vi "TableToArray(SubVI).vi"(11 "String in":string) -> (2 "Array":sgl[](array[numeric]))   [LabVIEW 2017, in "LV_Unicorn.lvlib"]
uses:
  LV_Unicorn.lvlib
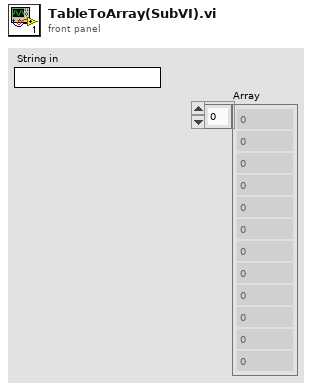
[diagram p1: front panel]
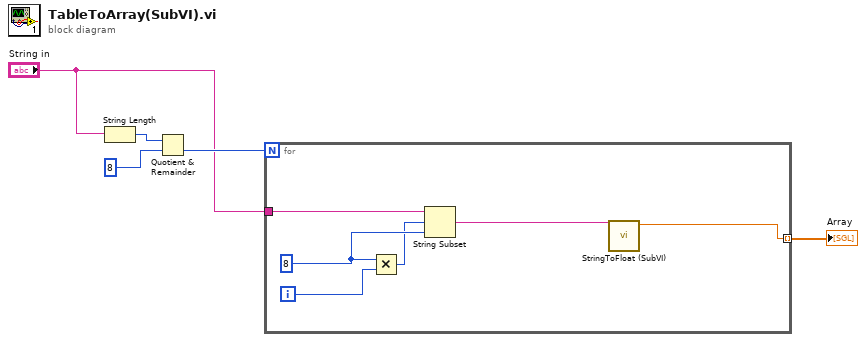
[diagram p0: block diagram]
diagram:
  n1 = String Length(string="String in") -> (length=w2:i32)
  n2 = Quotient & Remainder(x=w2, y=8) -> (floor(x/y)=w4:i32)  [unwired: 1 out]
  n3 = for {
    N: w4 -> [_]
    tunnel: "String in" -> [w11]
    tunnel: [w9] -> w5 mode=indexing
    i -> [w10]
    w7 = 8 ("length (rest)")
    n4 = Multiply(x=w7, y=w10) -> (x*y=w6:i32)
    n5 = String Subset(string=w11, offset (0)=w6, length (rest)=w7) -> (substring=w8:string)
    n6 = call "StringToFloat (SubVI).vi"("String in"=w8) -> ("Numeric"=w9:sgl)  [unwired: 10 in]
  }
  "Array" <- w5
